vi "Write AppInst.vi"(8 "error in (no error)":errorcluster, 10 "AppInst":refnum<vi>, 11 "Message Maker in":refnum<class "Message Scripter.lvclass">) -> (0 "error out":errorcluster, 3 "Message Maker out":refnum<class "Message Scripter.lvclass">)   [LabVIEW 2020, in "Message Maker.lvlib" / "Message Scripter.lvclass"]
uses:
  Message Scripter.lvclass
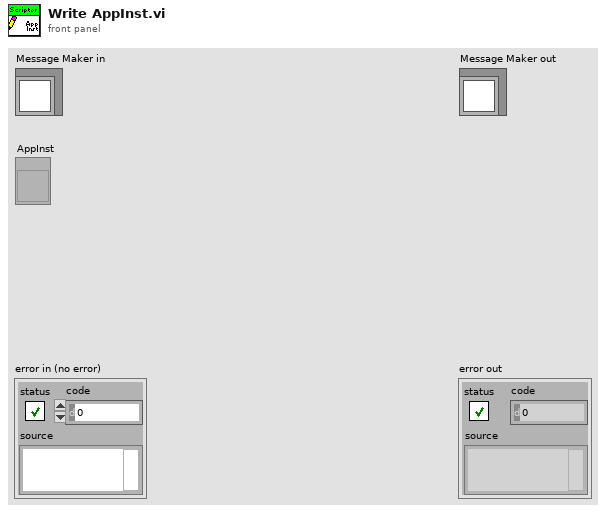
[diagram p1: front panel]
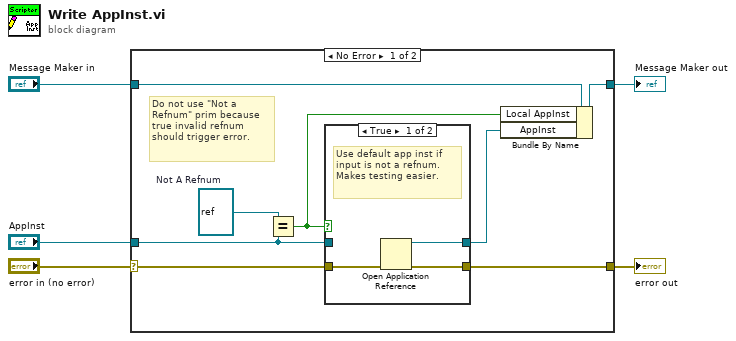
[diagram p0: block diagram]
diagram:
  n1 = case shown="No Error" "error in (no error)" {
    selector: "error in (no error)" -> [w8 w19]
    tunnel: [w9 w19] -> w4
    tunnel: [w12 w20] -> w2
    tunnel: "Message Maker in" -> [w13 w20]
    tunnel: "AppInst" -> [w7 _]
    frame No Error {
      w6 = refnum<vi> refnum  # Not A Refnum
      # "Do not use \"Not a Refnum\" prim because true invalid refnum should trigger error."
      n2 = Equal?(x=w6, y=w7) -> (x = y?=w11:bool)
      n3 = case shown="True" w11 {
        tunnel: w8 -> [w16 w18]
        tunnel: [w15 w18] -> w9
        tunnel: [w14 w17] -> w10
        tunnel: w7 -> [_ w17]
        frame True {
          # "Use default app inst if input is not a refnum. Makes testing easier."
          n4 = Open Application Reference(8:w16) -> (0:w15:errorcluster, 3:w14:refnum<vi>)  [unwired: 3 in]
        }
        frame False {
        }
      }
      n5 = Bundle By Name(cluster=w13, "Local AppInst"=w11, "AppInst"=w10) -> (w12:refnum<class "Message Scripter.lvclass">)
    }
    frame Error {
    }
  }
  "error out" <- w4
  "Message Maker out" <- w2
